vi "main.vi"(11 "Message Input":T1) -> (5 "Message Output":T1)   [LabVIEW 2025, in "Module 1.lvlib"]
uses:
  Module 1.lvlib
  <extravilib>/ChannelInstances/Event Messenger-t'Channel Messages.lvlib-Message Cluster.ctl'/))Channel.ctl
  Channel Messages/Message Cluster.ctl
  <extravilib>/ChannelInstances/Event Messenger-t'Channel Messages.lvlib-Message Cluster.ctl'/Event Data.ctl
  <extravilib>/ChannelInstances/Event Messenger-dbl/Event Data.ctl
  Module 1 Cases.ctl
  Module Main Cases.ctl
  80e217b9-4d7b-47f4-9f02-cca44f89b6ba.vi
  ded4d600-787e-431c-9f09-eae6f38a1613.vi
  9026f521-5d11-444e-8dfc-7e93337da711.vi
  3ecbbfb7-ecf9-4d68-a3d1-58c958038b39.vi
  178da06e-b036-45dc-94a7-9a73a3e7ae02.vi
  b7e3fb59-4668-43f0-bd5b-6f77558002f3.vi
  <vilib>/Utility/error.llb/Clear Errors.vi
  <extravilib>/ChannelInstances/Event Messenger-t'Channel Messages.lvlib-Message Cluster.ctl'/))Channel.vi
  <extravilib>/ChannelInstances/Messenger-c(t'Module 1 Cases.ctl',var)/Instantiate.vi
  <extravilib>/ChannelInstances/Tag-dbl/Instantiate.vi
  <extravilib>/ChannelInstances/Tag-bool/Instantiate.vi
  <extravilib>/ChannelInstances/Event Messenger-dbl/Instantiate.vi
  <extravilib>/ChannelInstances/Event Messenger-dbl/))Channel.vi
  <extravilib>/ChannelInstances/Messenger-c(t'Module 1 Cases.ctl',var)/Endpoint.vi
  Channel Messages/9242 error converting cmd string to case enum--error.vi
  <extravilib>/ChannelInstances/Tag-dbl/EndpointRead.vi
  <extravilib>/ChannelInstances/Tag-bool/EndpointRead.vi
  <extravilib>/ChannelInstances/Tag-dbl/Endpoint.vi
  <extravilib>/ChannelInstances/Tag-bool/Endpoint.vi
  <extravilib>/ChannelInstances/Messenger-c(t'Module 1 Cases.ctl',var).lvlib
  <extravilib>/ChannelInstances/Tag-dbl.lvlib
  <extravilib>/ChannelInstances/Event Messenger-t'Channel Messages.lvlib-Message Cluster.ctl'.lvlib
  <extravilib>/ChannelInstances/Event Messenger-dbl.lvlib
  Channel Messages/Channel Messages.lvlib
  <extravilib>/ChannelInstances/Tag-bool.lvlib
panel:
  in  "Init Button":bool
  out "Actual Position":dbl
  in  "Kill Button":bool
  in  "Stop Button":bool
  in  "Jog Target":dbl(slide) scale=0.0..100.0
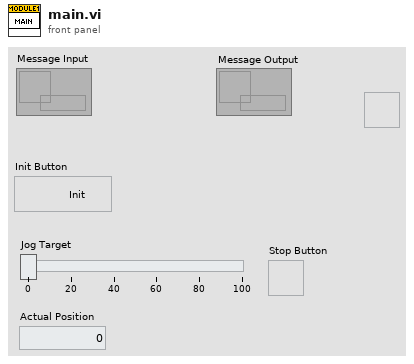
[diagram p1: front panel]
types:
  T1 = typedef "Event Messenger-t'Channel Messages.lvlib-Message Cluster.ctl'.lvlib/))Channel.ctl" = refnum<queue>
  T2 = cluster{"Message Input":refnum<event-registration>, "Jogger":refnum<event-registration>}
  T3 = typedef "Module 1 Cases.ctl" = enum16{"Kill", "Stop", "Init", "Jog"}
  T4 = typedef "Messenger-c(t'Module 1 Cases.ctl',var).lvlib/))Channel.ctl" = refnum<queue>
  T5 = typedef "Channel Messages.lvlib/Message Cluster.ctl" = cluster{"cmd":string, "data":variant}
  T6 = typedef "Module Main Cases.ctl" = enum16{"Error", "Log"}
  T7 = typedef "Tag-dbl.lvlib/))Channel.ctl" = refnum<queue>
  T8 = typedef "Tag-bool.lvlib/))Channel.ctl" = refnum<queue>
  T9 = typedef "Event Messenger-dbl.lvlib/))Channel.ctl" = refnum<queue>
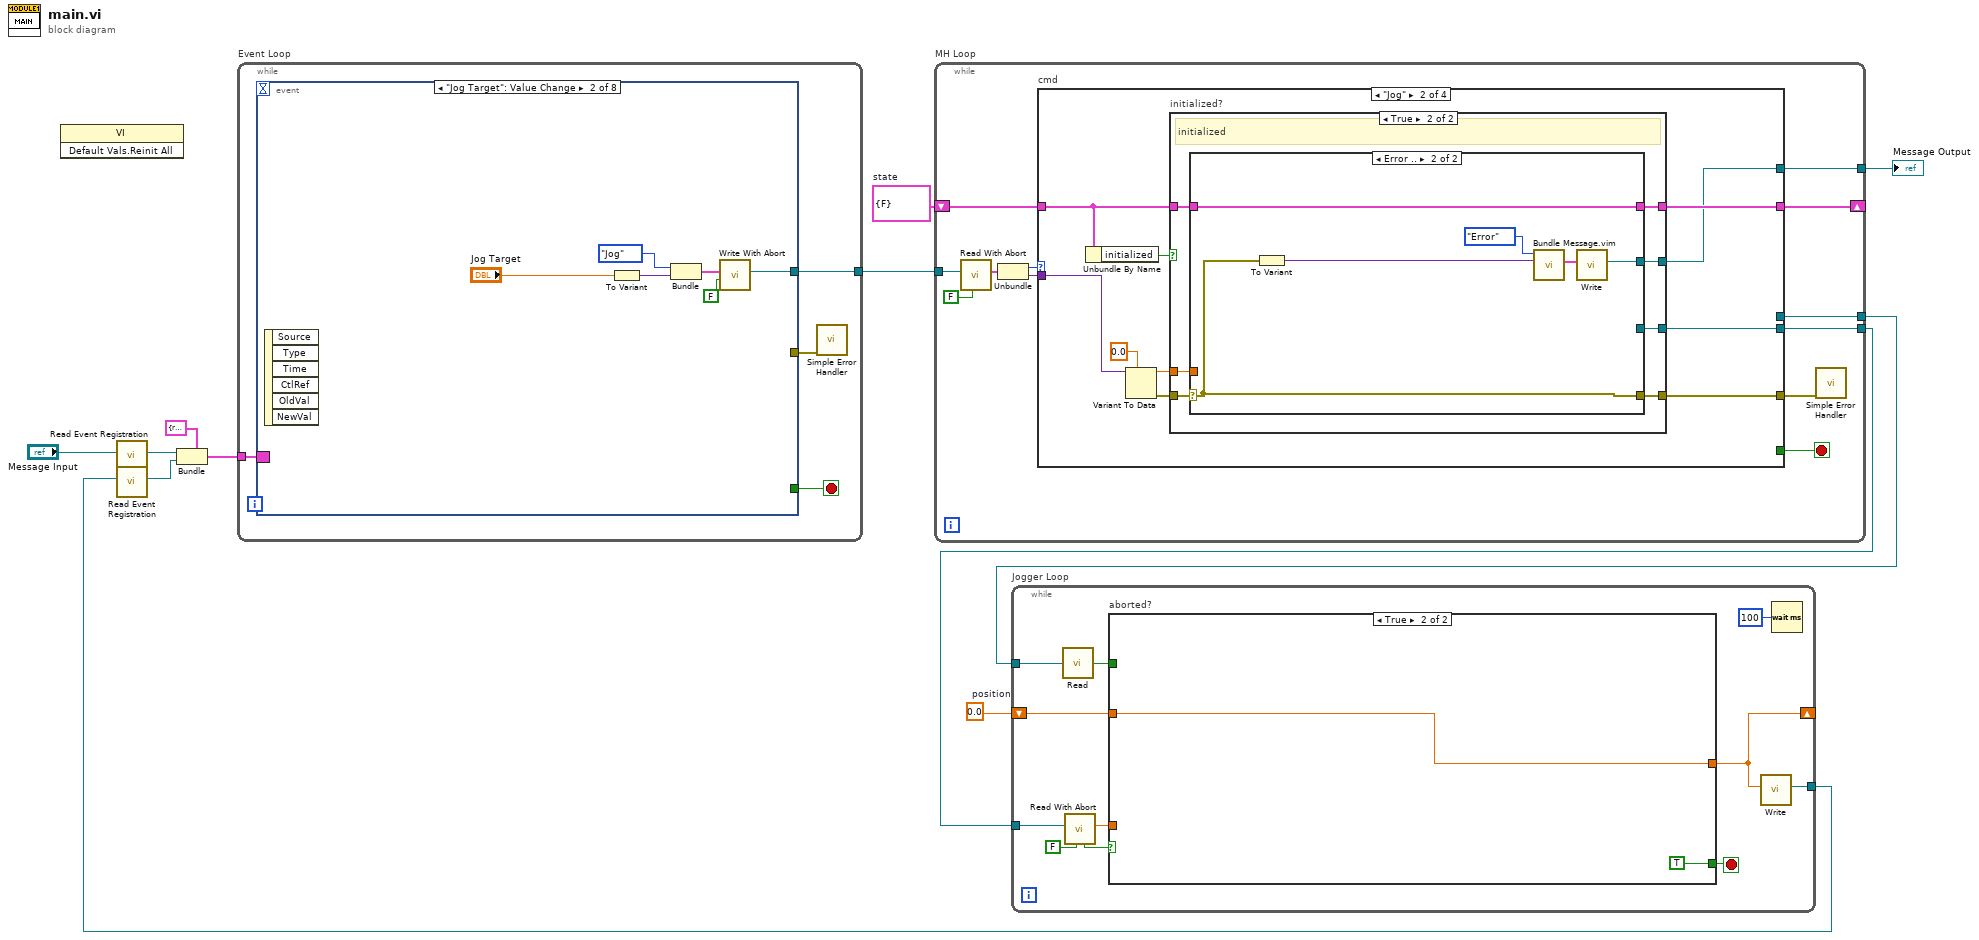
[diagram p0: block diagram]
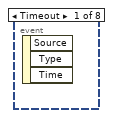
[diagram p2: hidden frame]
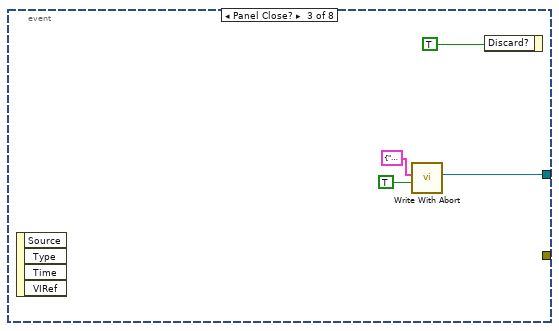
[diagram p3: hidden frame]
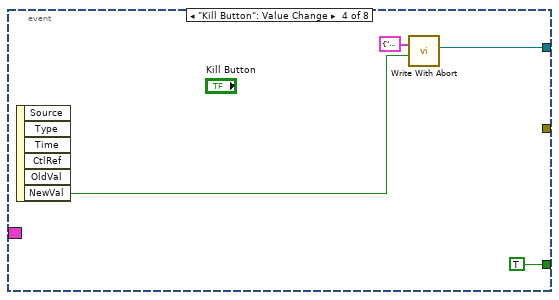
[diagram p4: hidden frame]
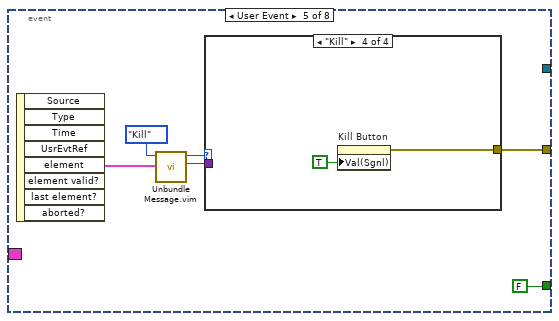
[diagram p5: hidden frame]
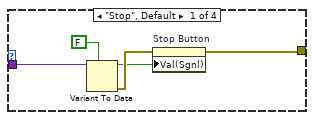
[diagram p6: hidden frame]
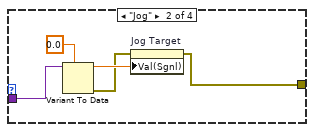
[diagram p7: hidden frame]
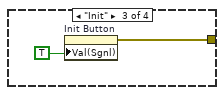
[diagram p8: hidden frame]
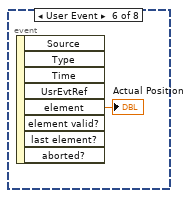
[diagram p9: hidden frame]
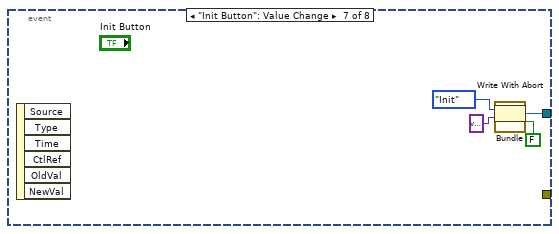
[diagram p10: hidden frame]
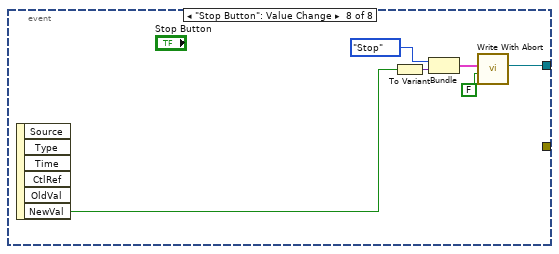
[diagram p11: hidden frame]
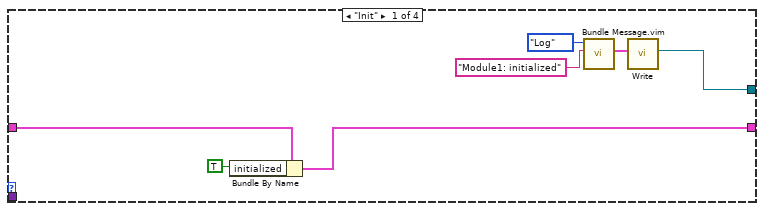
[diagram p12: hidden frame]
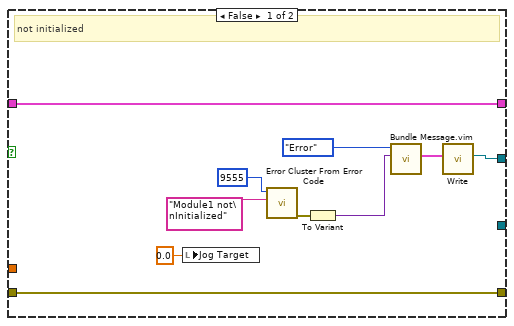
[diagram p13: hidden frame]
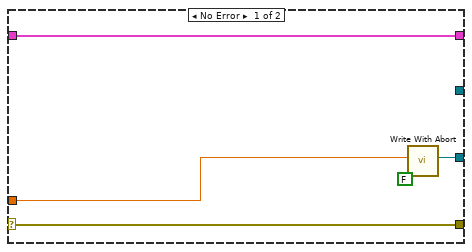
[diagram p14: hidden frame]
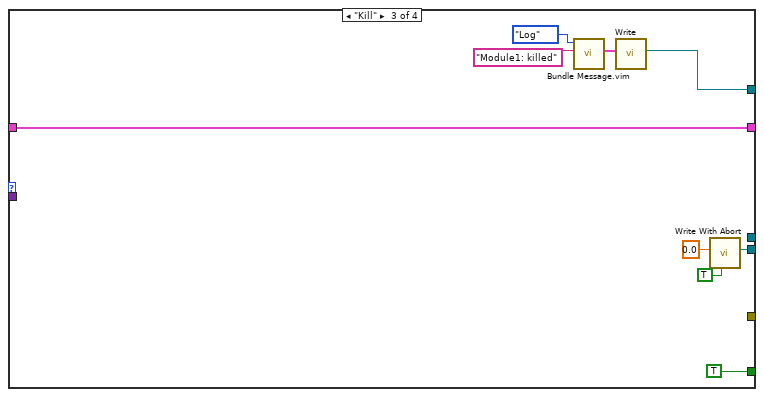
[diagram p15: hidden frame]
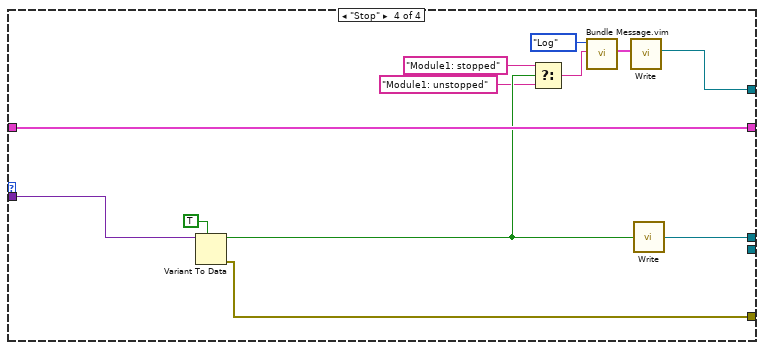
[diagram p16: hidden frame]
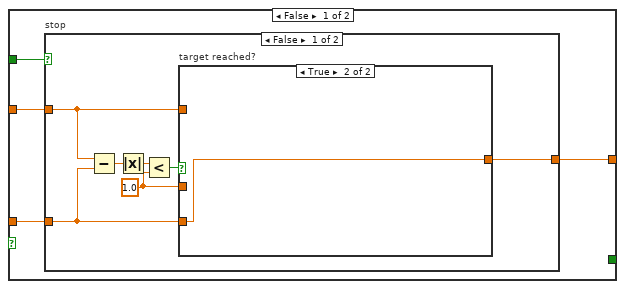
[diagram p17: hidden frame]
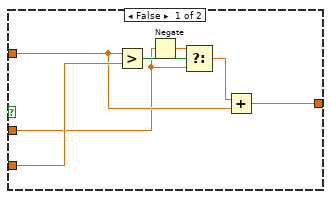
[diagram p18: hidden frame]
diagram:
  w2 = 0.0  # position
  w12 = cluster{"initialized":bool} {"initialized"=FALSE}  # state
  n1 = invoke class="VI" method="Default Vals.Reinit All"() -> ()  [unwired: 3 in, 3 out]
  n2 = call <extravilib>:"Read Event Registration.vi"("channel"="Message Input") -> ("event registration refnum"=w9:refnum<event-registration>)  [unwired: 10 in]
  n3 = call <extravilib>:"Read Event Registration.vi"("channel"=w8) -> ("event registration refnum"=w6:refnum<event-registration>)  [unwired: 10 in]
  n4 = Bundle(cluster=T2 {"Message Input"=refnum, "Jogger"=refnum}, "Message Input"=w9, "Jogger"=w6) -> (w7:T2)
  n5 = while "Event Loop" {
    tunnel: w7 -> [w15]
    tunnel: [w13] -> w1
    stop <- w14 stop-if-true
    n6 = event shown="[1] \"Jog Target\": Value Change" {
      selector: w15 -> [_ _ _ _ _ _ _ _]
      dyn-events: _ -> [_ _ _ _ _ _ _ _]
      timeout: _ -> [_ _ _ _ _ _ _ _]
      tunnel: [_ _ _ _ w35 _ _ _] -> w16
      tunnel: [_ _ _ TRUE FALSE _ _ _] -> w14
      tunnel: [_ w17 w23 w28 _ _ w52 w57] -> w13
      event Timeout {
        n7 = event-data() -> ()  [unwired: 1 in, 3 out]
      }
      event "Jog Target": Value Change {
        n8 = event-data() -> ()  [unwired: 1 in, 6 out]
        n9 = To Variant(anything="Jog Target") -> (Variant=w18:variant)
        n10 = Bundle("case"=Module_1_Cases."Jog", "Variant"=w18) -> (w21:cluster{"case":T3, "Variant":variant})  [unwired: 1 in]
        n11 = call <extravilib>:"Write With Abort.vi"("abort (F)"=FALSE, "element"=w21) -> ("channel"=w17:T4)  [unwired: 6 in, 3 out]
      }
      event Panel Close? {
        n12 = event-data() -> ()  [unwired: 1 in, 4 out]
        n13 = call <extravilib>:"Write With Abort.vi"("abort (F)"=TRUE, "element"=cluster{"Cmd":T3, "Data":variant} {"Cmd"=enum."Kill", "Data"=variant}) -> ("channel"=w23:T4)  [unwired: 6 in, 3 out]
        n14 = event-data("Discard?"=TRUE) -> ()  [unwired: 1 in, 1 out]
      }
      event "Kill Button": Value Change {
        n15 = event-data() -> ("NewVal"=w27:bool)  [unwired: 1 in, 5 out]
        n16 = call <extravilib>:"Write With Abort.vi"("abort (F)"=w27, "element"=cluster{"Cmd":T3, "Data":variant} {"Cmd"=enum."Kill", "Data"=variant}) -> ("channel"=w28:T4)  [unwired: 6 in, 3 out]
      }
      event User Event {
        n17 = event-data() -> ("element"=w36:T5)  [unwired: 1 in, 7 out]
        n18 = call "Unbundle Message.vim"("message"=w36, "cases type"=Module_1_Cases."Kill" ("Case")) -> ("data"=w31:variant, "case"=w32:T3)  [unwired: 7 in, 1 out]
        n19 = case shown="\"Kill\"" w32 {
          tunnel: w31 -> [w40 w46 _ _]
          tunnel: [w41 w42 w48 w50] -> w35
          frame "Stop", Default {
            n20 = Variant To Data(type=FALSE, Variant=w40) -> (data=w37:bool, error out=w38:errorcluster)  [unwired: 1 in]
            n21 = property on="Stop Button" class="Bool (strict)"(error in=w38, "Val(Sgnl)"=w37) -> (error out=w41:errorcluster)  [unwired: 1 in, 1 out]
          }
          frame "Jog" {
            n22 = Variant To Data(type=0.0, Variant=w46) -> (data=w44:dbl, error out=w43:errorcluster)  [unwired: 1 in]
            n23 = property on="Jog Target" class="Slide (strict)"(error in=w43, "Val(Sgnl)"=w44) -> (error out=w42:errorcluster)  [unwired: 1 in, 1 out]
          }
          frame "Init" {
            n24 = property on="Init Button" class="Bool"("Val(Sgnl)"=TRUE) -> (error out=w48:errorcluster)  [unwired: 2 in, 1 out]
          }
          frame "Kill" {
            n25 = property on="Kill Button" class="Bool (strict)"("Val(Sgnl)"=TRUE) -> (error out=w50:errorcluster)  [unwired: 2 in, 1 out]
          }
        }
      }
      event User Event {
        n26 = event-data() -> ("element"=→"Actual Position":dbl)  [unwired: 1 in, 7 out]
      }
      event "Init Button": Value Change {
        n27 = event-data() -> ()  [unwired: 1 in, 6 out]
        n28 = Bundle("Case"=Module_1_Cases."Init", variant) -> (w54:cluster{"Case":T3, variant})  [unwired: 1 in]
        n29 = call <extravilib>:"Write With Abort.vi"("abort (F)"=FALSE, "element"=w54) -> ("channel"=w52:T4)  [unwired: 6 in, 3 out]
      }
      event "Stop Button": Value Change {
        n30 = event-data() -> ("NewVal"=w59:bool)  [unwired: 1 in, 5 out]
        n31 = To Variant(anything=w59) -> (Variant=w58:variant)
        n32 = Bundle("case"=Module_1_Cases."Stop", "Variant"=w58) -> (w61:cluster{"case":T3, "Variant":variant})  [unwired: 1 in]
        n33 = call <extravilib>:"Write With Abort.vi"("abort (F)"=FALSE, "element"=w61) -> ("channel"=w57:T4)  [unwired: 6 in, 3 out]
      }
    }
    n34 = call <vilib>:"Simple Error Handler.vi"("error in (no error)"=w16) -> ()  [unwired: 4 in, 5 out]
  }
  n35 = while "MH Loop" {
    shift-right: [w72] -> _
    shift-left: w12 -> [w73]
    tunnel: [w69] -> w11
    tunnel: [w68] -> w4
    tunnel: [w67] -> w3
    tunnel: w1 -> [w66]
    stop <- w70 stop-if-true
    n36 = call <extravilib>:"Read With Abort.vi"("abort (F)"=FALSE, "channel"=w66) -> ("element"=w65:cluster{"Cmd":T3, "Data":variant})  [unwired: 6 in, 3 out]
    n37 = Unbundle(w65) -> ("Cmd"=w64:T3, "Data"=w74:variant)
    n38 = case "cmd" shown="\"Jog\"" w64 {
      tunnel: w74 -> [_ w91 _ w139]
      tunnel: w73 -> [w81 w89 w127 w140]
      tunnel: [w79 w88 w127 w140] -> w72
      tunnel: [_ w86 _ w137] -> w71
      tunnel: [_ _ TRUE _] -> w70
      tunnel: [w75 w84 w123 w132] -> w69
      tunnel: [_ _ _ w136] -> w68
      tunnel: [_ w82 w120 _] -> w67
      frame "Init" {
        n39 = Bundle By Name(cluster=w81, "initialized"=TRUE) -> (w79:cluster{"initialized":bool})
        n40 = call "Bundle Message.vim"("Data"="Module1: initialized", "Case"=Module_Main_Cases."Log") -> ("Message Cluster"=w76:T5)  [unwired: 9 in]
        n41 = call <extravilib>:"Write.vi"("element"=w76) -> ("channel"=w75:T1)  [unwired: 9 in, 1 out]
      }
      frame "Jog" {
        n42 = Unbundle By Name(w89) -> ("initialized"=w83:bool)
        n43 = Variant To Data(type=0.0, Variant=w91) -> (data=w87:dbl, error out=w85:errorcluster)  [unwired: 1 in]
        n44 = case "initialized?" shown="True" w83 {
          tunnel: w89 -> [w101 w106]
          tunnel: [w101 w105] -> w88
          tunnel: w87 -> [_ w102]
          tunnel: [w97 w107] -> w86
          tunnel: w85 -> [w97 w108]
          tunnel: [w93 w104] -> w84
          tunnel: [_ w103] -> w82
          frame False {
            # "not initialized"
            n45 = local write "Jog Target"(0.0) -> ()
            n46 = call <vilib>:"Error Cluster From Error Code.vi"("error message (\"\")"="Module1 not\nInitialized" ("error message (\"\")"), "error code (0)"=9555) -> ("error out"=w99:errorcluster)  [unwired: 7 in]
            n47 = To Variant(anything=w99) -> (Variant=w95:variant)
            n48 = call "Bundle Message.vim"("Data"=w95, "Case"=Module_Main_Cases."Error") -> ("Message Cluster"=w94:T5)  [unwired: 9 in]
            n49 = call <extravilib>:"Write.vi"("element"=w94) -> ("channel"=w93:T1)  [unwired: 9 in, 1 out]
          }
          frame True {
            # "initialized"
            n50 = case shown="Error .." w108 {
              selector: w108 -> [w113 w118]
              tunnel: [w113 w118] -> w107
              tunnel: w106 -> [w109 w119]
              tunnel: [w109 w119] -> w105
              tunnel: [_ w114] -> w104
              tunnel: [w112 _] -> w103
              tunnel: w102 -> [w110 _]
              frame No Error {
                n51 = call <extravilib>:"Write With Abort.vi"("abort"=FALSE, "element"=w110) -> ("channel"=w112:T7)  [unwired: 7 in, 2 out]
              }
              frame Error {
                n52 = To Variant(anything=w118) -> (Variant=w116:variant)
                n53 = call "Bundle Message.vim"("Data"=w116, "Case"=Module_Main_Cases."Error") -> ("Message Cluster"=w115:T5)  [unwired: 9 in]
                n54 = call <extravilib>:"Write.vi"("element"=w115) -> ("channel"=w114:T1)  [unwired: 9 in, 1 out]
              }
            }
          }
        }
      }
      frame "Kill" {
        n55 = call "Bundle Message.vim"("Data"="Module1: killed", "Case"=Module_Main_Cases."Log") -> ("Message Cluster"=w124:T5)  [unwired: 9 in]
        n56 = call <extravilib>:"Write.vi"("element"=w124) -> ("channel"=w123:T1)  [unwired: 9 in, 1 out]
        n57 = call <extravilib>:"Write With Abort.vi"("abort"=TRUE, "element"=0.0) -> ("channel"=w120:T7)  [unwired: 7 in, 2 out]
      }
      frame "Stop" {
        n58 = Variant To Data(type=TRUE, Variant=w139) -> (data=w130:bool, error out=w137:errorcluster)  [unwired: 1 in]
        n59 = Select(t="Module1: stopped", s=w130, f="Module1: unstopped") -> (s? t:f=w131:string)
        n60 = call "Bundle Message.vim"("Data"=w131, "Case"=Module_Main_Cases."Log") -> ("Message Cluster"=w133:T5)  [unwired: 9 in]
        n61 = call <extravilib>:"Write.vi"("element"=w133) -> ("channel"=w132:T1)  [unwired: 9 in, 1 out]
        n62 = call <extravilib>:"Write.vi"("element"=w130) -> ("channel"=w136:T8)  [unwired: 1 out]
      }
    }
    n63 = call <vilib>:"Simple Error Handler.vi"("error in (no error)"=w71) -> ()  [unwired: 4 in, 5 out]
  }
  "Message Output" <- w11
  n64 = while "Jogger Loop" {
    shift-right: [w142] -> _
    shift-left: w2 -> [w151]
    tunnel: [w149] -> w8
    tunnel: w4 -> [w144]
    tunnel: w3 -> [w148]
    stop <- w150 stop-if-true
    n65 = call <extravilib>:"Read.vi"("channel"=w144) -> ("element"=w143:bool)  [unwired: 1 in, 1 out]
    n66 = call <extravilib>:"Read With Abort.vi"("abort"=FALSE, "channel"=w148) -> ("element"=w146:dbl, "aborted?"=w145:bool)  [unwired: 7 in, 1 out]
    n67 = case "aborted?" shown="True" w145 {
      tunnel: w151 -> [w155 w172]
      tunnel: [w154 w172] -> w142
      tunnel: [_ TRUE] -> w150
      tunnel: w146 -> [w153 _]
      tunnel: w143 -> [w152 _]
      frame False {
        n68 = case "stop" shown="False" w152 {
          tunnel: w155 -> [w160 w171]
          tunnel: [w162 w171] -> w154
          tunnel: w153 -> [w161 _]
          frame False {
            w156 = 1.0 ("y")
            n69 = Subtract(x=w160, y=w161) -> (x-y=w159:dbl)
            n70 = Absolute Value(x=w159) -> (abs(x)=w158:dbl)
            n71 = Less?(x=w158, y=w156) -> (x < y?=w157:bool)
            n72 = case "target reached?" shown="True" w157 {
              tunnel: [w165 w170] -> w162
              tunnel: w161 -> [w169 w170]
              tunnel: w160 -> [w167 _]
              tunnel: w156 -> [w164 _]
              frame False {
                n73 = Greater?(x=w167, y=w169) -> (0:w168:bool)
                n74 = Negate(x=w164) -> (-x=w163:dbl)
                n75 = Select(t=w163, s=w168, f=w164) -> (s? t:f=w166:dbl)
                n76 = Add(x=w166, y=w167) -> (x+y=w165:dbl)
              }
              frame True {
              }
            }
          }
          frame True {
          }
        }
      }
      frame True {
      }
    }
    n77 = call <extravilib>:"Write.vi"("element"=w142) -> ("channel"=w149:T9)  [unwired: 9 in, 1 out]
    n78 = Wait (ms)(milliseconds to wait=u32 100) -> ()  [unwired: 1 out]
  }
